vi "OFFINISH_compare.vi"(8 "errin":errorcluster, 9 "PlcFrame":string, 10 "étage":string, 11 "OFenC":string) -> (0 "errout":errorcluster, 1 "OFEnC":string caption="OF en cours coté Automate", 2 "L2T":T1, 3 "MB":string)   [LabVIEW 2020]
uses:
  <vilib>/Utility/config.llb/Write Key (String).vi
  <vilib>/Utility/config.llb/NI_LVConfig.lvlib
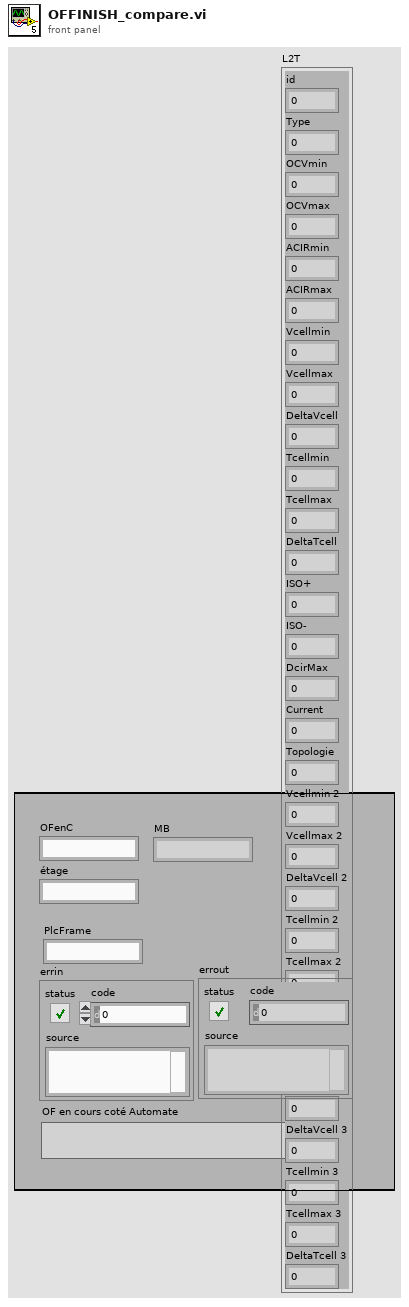
[diagram p1: front panel]
types:
  T1 = cluster{"id":dbl, "Type":dbl, "OCVmin":dbl, "OCVmax":dbl, "ACIRmin":dbl, "ACIRmax":dbl, "Vcellmin":dbl, "Vcellmax":dbl, "DeltaVcell":dbl, "Tcellmin":dbl, "Tcellmax":dbl, "DeltaTcell":dbl, "ISO+":dbl, "ISO-":dbl, "DcirMax":dbl, "Current":dbl, "Topologie":dbl, "Vcellmin 2":dbl, "Vcellmax 2":dbl, "DeltaVcell 2":dbl, "Tcellmin 2":dbl, "Tcellmax 2":dbl, "DeltaTcell 2":dbl, "Vcellmin 3":dbl, "Vcellmax 3":dbl, "DeltaVcell 3":dbl, "Tcellmin 3":dbl, "Tcellmax 3":dbl, "DeltaTcell 3":dbl}
  T2 = typedef "NI_LVConfig.lvlib/Config Data RefNum.ctl" = refnum<k1>
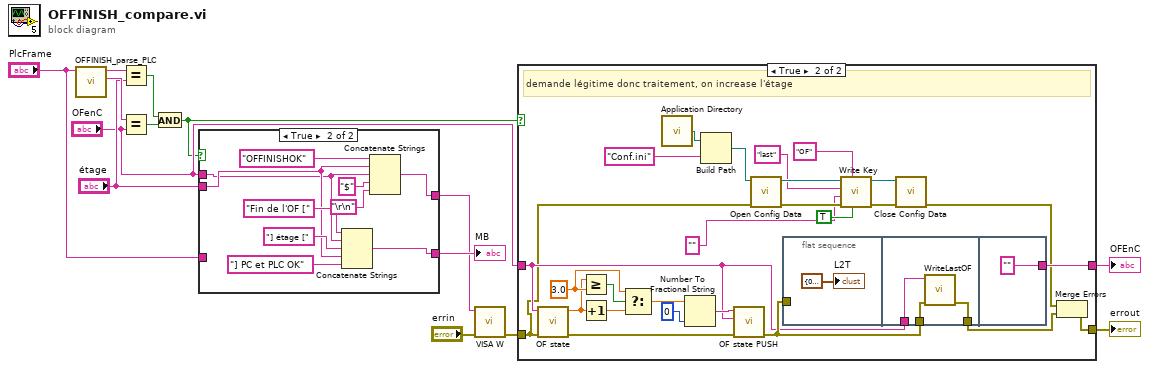
[diagram p0: block diagram]
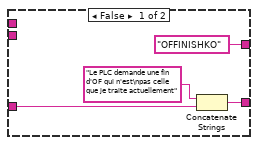
[diagram p3: hidden frame]
diagram:
  n1 = call "OFFINISH_parse_PLC.vi"("String"="PlcFrame") -> ("OF"=w11:string, "étage"=w10:string)  [unwired: 9 in]
  n2 = Equal?(x=w10, y="étage") -> (x = y?=w13:bool)
  n3 = Equal?(x=w11, y="OFenC") -> (x = y?=w12:bool)
  n4 = And(x=w13, y=w12) -> (x .and. y?=w2:bool)
  n5 = case shown="True" w2 {
    tunnel: [w18 w25] -> w14
    tunnel: "OFenC" -> [_ w19]
    tunnel: "étage" -> [_ w21]
    tunnel: "PlcFrame" -> [w16 _]
    tunnel: ["OFFINISHKO" w20] -> w6
    frame False {
      n6 = Concatenate Strings("Le PLC demande une fin d'OF qui n'est\npas celle que je traite actuellement" ("string"), w16) -> (w18:string)
    }
    frame True {
      n7 = Concatenate Strings("Fin de l'OF [" ("MSG"), w19, "] étage [" ("string"), w21, "] PC et PLC OK" ("string")) -> (w25:string)
      n8 = Concatenate Strings("OFFINISHOK" ("buffer d'écriture"), w21, w19, "$" ("string"), "\r\n") -> (w20:string)
    }
  }
  "MB" <- w14
  n9 = call "VISA W.vi"("errin"="errin", "Chaîne"=w6) -> ("errout"=w7:errorcluster)  [unwired: 9 in]
  n10 = case shown="True" w2 {
    tunnel: w7 -> [w30 w35]
    tunnel: "OFenC" -> [w29 w47]
    tunnel: [w30 w32] -> w3
    tunnel: [w29 w46] -> w1
    frame False {
    }
    frame True {
      w51 = 3.0 ("y")
      # "demande légitime donc traitement, on increase l'étage"
      n11 = call "OF state.vi"("errin"=w35, "OF"=w47) -> ("error out"=w55:errorcluster, "number dbl"=w50:dbl)  [unwired: 7 in, 1 out]
      n12 = Greater Or Equal? ("Supérieur ou égal ?")(x=w50, y=w51) -> (x >= y?=w52:bool)
      n13 = Increment(x=w50) -> (x+1=w49:dbl)
      n14 = Select(t=w51, s=w52, f=w49) -> (s? t:f=w48:dbl)
      n15 = call <vilib>:"Application Directory.vi"() -> ("Application Directory"=w43:path)
      n16 = Number To Fractional String ("Nombre en chaîne fractionnaire")(number=w48, precision (6)=i16 0 ("précision (6)")) -> (F-format string=w54:string)  [unwired: 2 in]
      n17 = Build Path ("Composer un chemin")(base path=w43, name or relative path="Conf.ini") -> (appended path=w42:path)
      n18 = call "OF state PUSH.vi"("errin"=w55, "OF"=w47, "result"=w54) -> ("error out"=w53:errorcluster)  [unwired: 8 in]
      n19 = call <vilib>:"Open Config Data.vi"("error in (no error)"=w35, "configuration file path"=w42) -> ("error out"=w44:errorcluster, "refnum"=w41:T2)  [unwired: 7 in, 1 out]
      n20 = flat-sequence {
        tunnel: w53 -> [_]
        tunnel: w53 -> [w60]
        tunnel: [w59] -> w34
        tunnel: w47 -> [w58]
        tunnel: [""] -> w46
        frame #0 {
          "L2T" <- T1 {"id"=0.0, "Type"=0.0, "OCVmin"=0.0, "OCVmax"=0.0, "ACIRmin"=0.0, "ACIRmax"=0.0, "Vcellmin"=0.0, "Vcellmax"=0.0, "DeltaVcell"=0.0, "Tcellmin"=0.0, "Tcellmax"=0.0, "DeltaTcell"=0.0, "ISO+"=0.0, "ISO-"=0.0, "DcirMax"=0.0, "Current"=0.0, "Topologie"=0.0, "Vcellmin 2"=0.0, "Vcellmax 2"=0.0, "DeltaVcell 2"=0.0, "Tcellmin 2"=0.0, "Tcellmax 2"=0.0, "DeltaTcell 2"=0.0, "Vcellmin 3"=0.0, "Vcellmax 3"=0.0, "DeltaVcell 3"=0.0, "Tcellmin 3"=0.0, "Tcellmax 3"=0.0, "DeltaTcell 3"=0.0} ("L2T")
        }
        frame #1 {
          n21 = call "WriteLastOF.vi"("errin"=w60, "OF to save"=w58) -> ("errout"=w59:errorcluster)  [unwired: 9 in]
        }
        frame #2 {
        }
      }
      n22 = call-poly <vilib>:"Write Key.vi"("write raw string? (F)"=TRUE, "section"="OF", "error in (no error)"=w44, "value"="", "key"="last", "refnum"=w41) -> ("error out"=w45:errorcluster, "refnum out"=w40:T2)  [unwired: 3 in, 1 out]
      n23 = call <vilib>:"Close Config Data.vi"("error in (no error)"=w45, "refnum"=w40) -> ("error out"=w33:errorcluster)  [unwired: 8 in, 1 out]
      n24 = Merge Errors(w33, w34) -> (w32:errorcluster)
    }
  }
  "errout" <- w3
  "OFEnC" <- w1
